vi "DC_settings.vi"(0 "ENABLE":bool, 1 "Select Range":string, 2 "Voltage Limit [V]":dbl, 3 "Current Limit [A]":dbl, 4 "E3631a address":string="2") -> ()   [LabVIEW 2019]
panel:
  # "DEBUG"
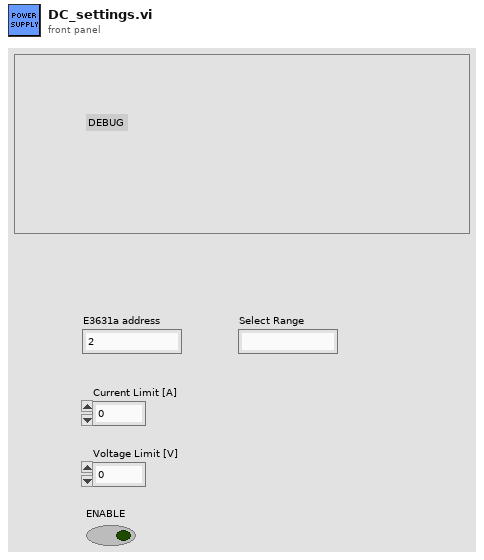
[diagram p1: front panel]
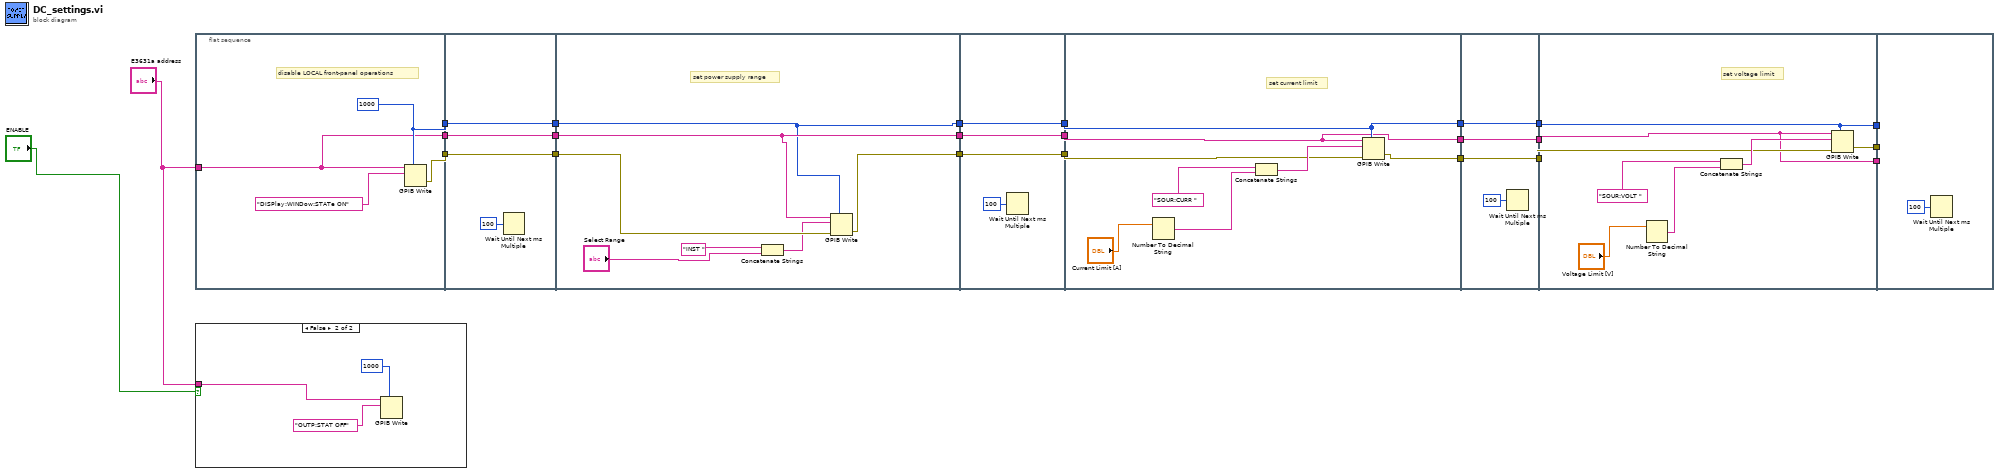
[diagram p0: block diagram]
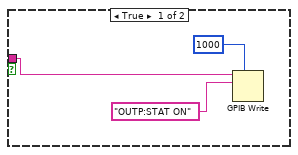
[diagram p2: hidden frame]
diagram:
  n1 = flat-sequence {
    tunnel: [w26] -> w23
    tunnel: [w24] -> w22
    tunnel: [w25] -> w21
    tunnel: "E3631a address" -> [w24]
    tunnel: w23 -> [w31]
    tunnel: [w31] -> w20
    tunnel: w22 -> [w30]
    tunnel: [w30] -> w19
    tunnel: w21 -> [w29]
    tunnel: [w29] -> w18
    tunnel: w20 -> [w37]
    tunnel: [w37] -> w17
    tunnel: w19 -> [w38]
    tunnel: w18 -> [w35]
    tunnel: [w36] -> w16
    tunnel: [w38] -> w15
    tunnel: w17 -> [w42]
    tunnel: [w42] -> w14
    tunnel: w16 -> [w41]
    tunnel: [w41] -> w13
    tunnel: w15 -> [w40]
    tunnel: [w40] -> w12
    tunnel: w14 -> [w46]
    tunnel: w13 -> [w47]
    tunnel: [w46] -> w11
    tunnel: [w45] -> w10
    tunnel: [w44] -> w9
    tunnel: w12 -> [w45]
    tunnel: w11 -> [w54]
    tunnel: [w54] -> w8
    tunnel: w10 -> [w53]
    tunnel: [w53] -> w7
    tunnel: w9 -> [w52]
    tunnel: [w52] -> w6
    tunnel: w8 -> [w58]
    tunnel: w7 -> [w57]
    tunnel: w6 -> [w59]
    tunnel: [w58] -> w3
    tunnel: [w57] -> w4
    tunnel: [w56] -> w5
    tunnel: w5 -> [_]
    tunnel: w4 -> [_]
    tunnel: w3 -> [_]
    frame #0 {
      w26 = 1000 ("timeout ms (488.2 global)")
      # "disable LOCAL front-panel operations"
      n2 = GPIB Write(0:w24, 1:"DISPlay:WINDow:STATe ON" ("data"), 4:w26) -> (6:w25:errorcluster)  [unwired: 2 in, 1 out]
    }
    frame #1 {
      n3 = Wait Until Next ms Multiple(millisecond multiple=u32 100) -> ()  [unwired: 1 out]
    }
    frame #2 {
      # "set power supply range"
      n4 = Concatenate Strings("INST " ("data"), "Select Range") -> (w34:string)
      n5 = GPIB Write(0:w38, 1:w34, 3:w35, 4:w37) -> (6:w36:errorcluster)  [unwired: 1 in, 1 out]
    }
    frame #3 {
      n6 = Wait Until Next ms Multiple(millisecond multiple=u32 100) -> ()  [unwired: 1 out]
    }
    frame #4 {
      # "set current limit"
      n7 = Number To Decimal String(number="Current Limit [A]") -> (decimal integer string=w48:string)  [unwired: 1 in]
      n8 = Concatenate Strings("SOUR:CURR " ("data"), w48) -> (w49:string)
      n9 = GPIB Write(0:w45, 1:w49, 3:w47, 4:w46) -> (6:w44:errorcluster)  [unwired: 1 in, 1 out]
    }
    frame #5 {
      n10 = Wait Until Next ms Multiple(millisecond multiple=u32 100) -> ()  [unwired: 1 out]
    }
    frame #6 {
      # "set voltage limit"
      n11 = Number To Decimal String(number="Voltage Limit [V]") -> (decimal integer string=w60:string)  [unwired: 1 in]
      n12 = Concatenate Strings("SOUR:VOLT " ("data"), w60) -> (w61:string)
      n13 = GPIB Write(0:w57, 1:w61, 3:w59, 4:w58) -> (6:w56:errorcluster)  [unwired: 1 in, 1 out]
    }
    frame #7 {
      n14 = Wait Until Next ms Multiple(millisecond multiple=u32 100) -> ()  [unwired: 1 out]
    }
  }
  n15 = case shown="False" "ENABLE" {
    tunnel: "E3631a address" -> [w65 w68]
    frame True {
      n16 = GPIB Write(0:w65, 1:"OUTP:STAT ON" ("data"), 4:1000 ("timeout ms (488.2 global)")) -> ()  [unwired: 2 in, 2 out]
    }
    frame False {
      n17 = GPIB Write(0:w68, 1:"OUTP:STAT OFF" ("data"), 4:1000) -> ()  [unwired: 2 in, 2 out]
    }
  }
